vi "Read Response.vi"(8 "error in (no error)":errorcluster, 9 "timeout in ms (0)":i32, 11 "Interface in":refnum<class "Interface.lvclass">) -> (0 "error out":errorcluster, 1 "timed out?":bool, 2 "response":T1, 3 "Interface out":refnum<class "Interface.lvclass">, 4 "# elements":u32)   [LabVIEW 2017, in "DSF Core.lvlib" / "Interface.lvclass"]
uses:
  Interface.lvclass
  RT FIFO Data 16B.ctl
  RT FIFO Payload 16B.ctl
  Interface.lvclass/Interface.ctl
  Response Timeout.vi
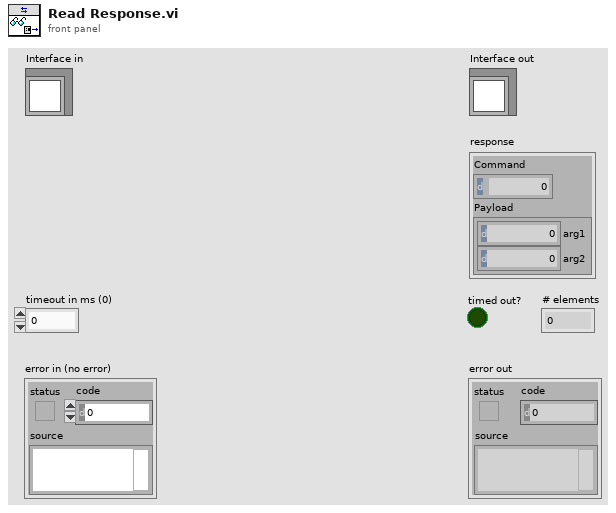
[diagram p1: front panel]
types:
  T1 = typedef "DSF Core.lvlib/Interface.lvclass/RT FIFO Data 16B.ctl" = cluster{"Command":u8, "Payload":T2}
  T2 = typedef "DSF Core.lvlib/Interface.lvclass/RT FIFO Payload 16B.ctl" = cluster{"arg1":u64, "arg2":u64}
  T3 = typedef "DSF Core.lvlib/FIFO Flags.ctl" = cluster{"Infinite Timeouts":bool}
  T4 = typedef "DSF Core.lvlib/Interface.lvclass/RT FIFO Ref 16B.ctl" = refnum<k33>
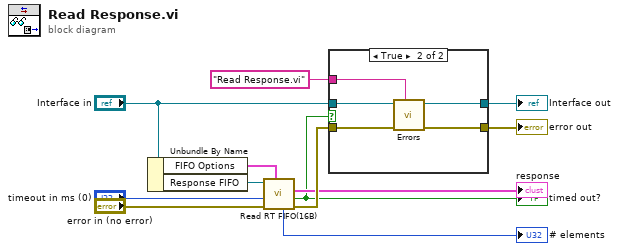
[diagram p0: block diagram]
diagram:
  n1 = Unbundle By Name("Interface in") -> ("FIFO Options"=w1:T3, "Response FIFO"=w2:T4)
  n2 = call "Read RT FIFO(16B).vi"("FIFO Options"=w1, "error in (no error)"="error in (no error)", "timeout in ms (0)"="timeout in ms (0)", "RT FIFO in"=w2) -> ("error out"=w8:errorcluster, "empty?"=w4:bool, "element out"=→"response":T1, "# elements"=→"# elements":u32)  [unwired: 3 in, 1 out]
  "timed out?" <- w4
  n3 = case shown="True" w4 {
    tunnel: "Interface in" -> [w14 w19]
    tunnel: [w14 w18] -> w9
    tunnel: [w13 w17] -> w7
    tunnel: w8 -> [w13 w16]
    tunnel: "Read Response.vi" ("error source vi name") -> [_ w15]
    frame False {
    }
    frame True {
      n4 = call-poly "Errors.vi"("error source vi name"=w15, "error in (no error)"=w16, "Interface in"=w19) -> ("error out"=w17:errorcluster, "Interface out"=w18:refnum<class "Interface.lvclass">)  [unwired: 7 in]
    }
  }
  "error out" <- w7
  "Interface out" <- w9
